vi "30 GPS Time Fetch (2017).vi"() -> ()   [LabVIEW 2017]
panel:
  out "GPS Time Error":dbl format="%.6f"
  out "CPU Time Error":dbl format="%.6f"
  out "GPS Date":string
  out "GPS Time":string
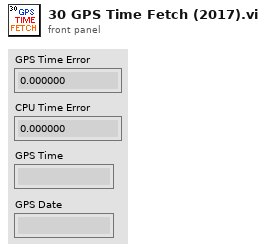
[diagram p1: front panel]
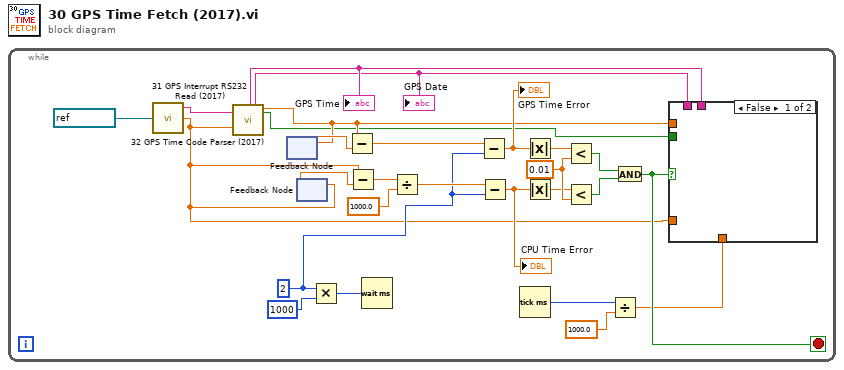
[diagram p0: block diagram]
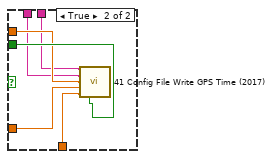
[diagram p2: hidden frame]
diagram:
  n1 = while {
    stop <- w15 stop-if-true
    w18 = 0.01 ("y")
    w19 = u32 2 ("milliseconds to wait")
    n2 = call "31 GPS Interrupt RS232 Read (2017).vi"("Comm Port"=refnum<visa-resource-name> "COM3") -> ("GPS Time Code"=w4:string, "CPU Time"=w3:dbl)  [unwired: 4 in, 1 out]
    n3 = call "32 GPS Time Code Parser (2017).vi"("GPS Time Code"=w4, "CPU Time In"=w3) -> ("GPS Time"=w6:string, "GPS Date"=w5:string, "Labview Time"=w2:dbl, "GPS Lock"=w1:bool)  [unwired: 6 in, 8 out]
    "GPS Date" <- w5
    "GPS Time" <- w6
    n4 = feedback-in #1(w2) -> ()
    n5 = feedback #1() -> (w26:dbl)  [unwired: 1 in]
    n6 = feedback-in #2(w3) -> ()
    n7 = feedback #2() -> (w27:dbl)  [unwired: 1 in]
    n8 = Multiply(x=w19, y=u32 1000) -> (x*y=w23:u32)
    n9 = Subtract(x=w2, y=w26) -> (x-y=w21:dbl)
    n10 = Subtract(x=w3, y=w27) -> (x-y=w25:dbl)
    n11 = Wait (ms)(milliseconds to wait=w23) -> ()  [unwired: 1 out]
    n12 = Divide(x=w25, y=1000.0) -> (x/y=w20:dbl)
    n13 = Subtract(x=w21, y=w19) -> (x-y=w11:dbl)
    "GPS Time Error" <- w11
    n14 = Subtract(x=w20, y=w19) -> (x-y=w14:dbl)
    "CPU Time Error" <- w14
    n15 = Tick Count (ms)() -> (millisecond timer value=w9:u32)
    n16 = Absolute Value(x=w11) -> (abs(x)=w12:dbl)
    n17 = Absolute Value(x=w14) -> (abs(x)=w13:dbl)
    n18 = Less?(x=w12, y=w18) -> (x < y?=w17:bool)
    n19 = Less?(x=w13, y=w18) -> (x < y?=w16:bool)
    n20 = Divide(x=w9, y=1000.0) -> (x/y=w8:dbl)
    n21 = And(x=w17, y=w16) -> (x .and. y?=w15:bool)
    n22 = case shown="False" w15 {
      tunnel: w2 -> [_ w30]
      tunnel: w3 -> [_ w31]
      tunnel: w6 -> [_ w28]
      tunnel: w5 -> [_ w29]
      tunnel: w8 -> [_ w32]
      tunnel: w1 -> [_ w33]
      frame False {
      }
      frame True {
        n23 = call "41 Config File Write GPS Time (2017).vi"("GPS Time"=w28, "GPS Date"=w29, "Labview Time"=w30, "CPU Time"=w31, "Tick Count"=w32, "GPS Lock"=w33) -> ()  [unwired: 10 in]
      }
    }
  }
